vi "Compute_the_given_expression_2.vi"() -> ()   [LabVIEW 2020]
uses:
  <vilib>/express/express arith-compare/Formula/XNode/ExpressFormulaBlockNode.xnode
panel:
  out "Using Express Formula":dbl
  out "Using Expression Nodes":dbl
  in  "X1":dbl
  out "Using Regular Functions":dbl
  # "Compute the expressions(X1+2)*log(X1) using Functions, Expression Node \nand Express Formula for the given inputs X1"
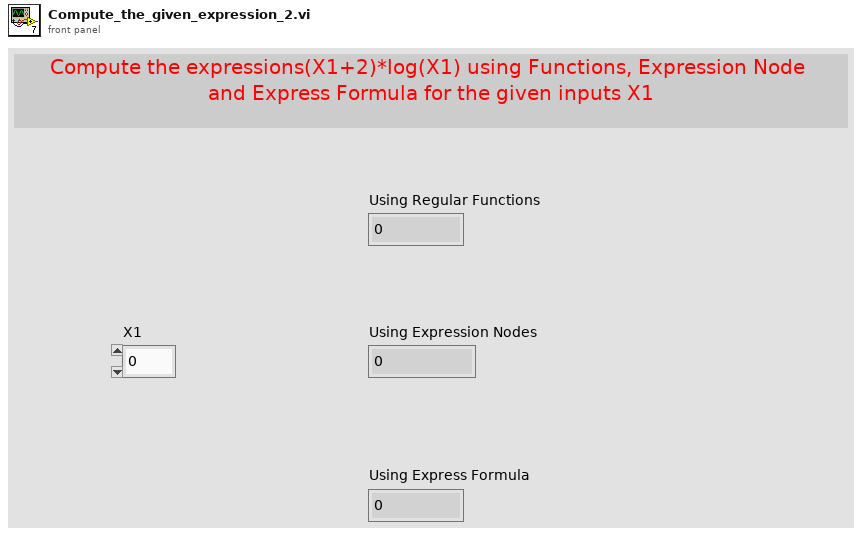
[diagram p1: front panel]
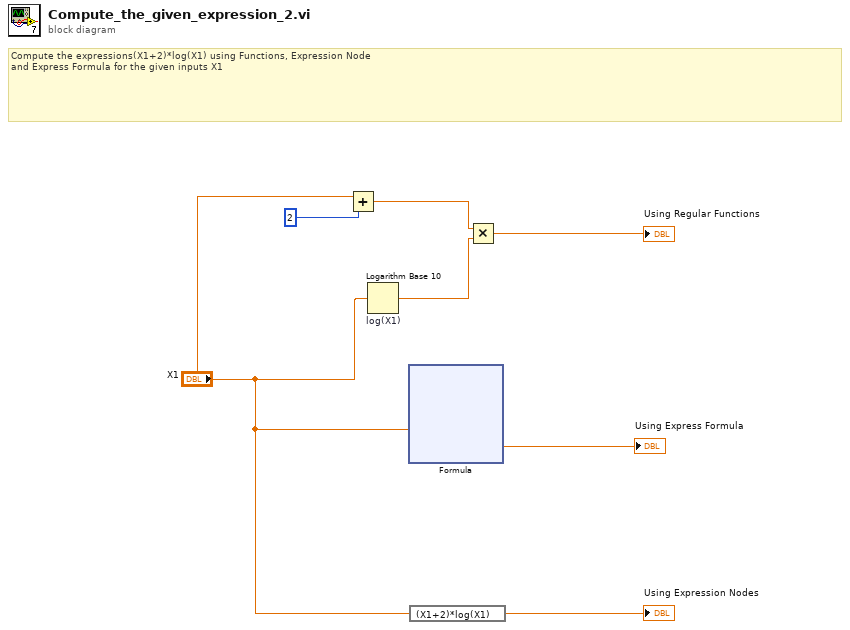
[diagram p0: block diagram]
diagram:
  # "Compute the expressions(X1+2)*log(X1) using Functions, Expression Node \nand Express Formula for the given inputs X1"
  n1 = Add(x="X1", y=2) -> (x+y=w7:dbl)
  n2 = Logarithm Base 10 "log(X1)"(1:"X1") -> (0:w5:dbl)
  n3 = xnode "Formula"("X1"="X1") -> ("Result"=→"Using Express Formula":dbl)  [unwired: 1 in, 1 out]
  n4 = expression code="(X1+2)*log(X1)"("X1") -> (→"Using Expression Nodes":dbl)
  n5 = Multiply(x=w7, y=w5) -> (x*y=→"Using Regular Functions":dbl)
